vi "TDMS File Viewer.vi"   [LabVIEW 2014]
panel:
  # "Run this VI to launch a TDMS File Viewer."
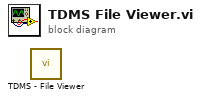
[diagram p0: block diagram]
diagram:
  n1 = call <vilib>:"TDMS - File Viewer.vi"() -> ()  [unwired: 6 in, 2 out]
